vi "ReadAttributeTest.vi"() -> ()   [LabVIEW 2009]
uses:
  tango_lv8/tango_vi.llb/ReadDoubleSpectrumAttribute.vi
  tango_lv8/tango_vi.llb/ReadDoubleScalarAttribute.vi
  tango_lv8/tango_vi.llb/ReadLongScalarAttribute.vi
  tango_lv8/tango_vi.llb/ReadLongSpectrumAttribute.vi
  tango_lv8/tango_vi.llb/ReadShortSpectrumAttribute.vi
  tango_lv8/tango_vi.llb/ReadShortScalarAttribute.vi
  tango_lv8/tango_vi.llb/ReadShortImageAttribute.vi
  tango_lv8/tango_vi.llb/ReadLongImageAttribute.vi
  tango_lv8/tango_vi.llb/ReadDoubleImageAttribute.vi
  tango_lv8/tango_vi.llb/ReadStringAttribute.vi
panel:
  out "?":string
  out "?":bool
  out "?":string
  out "?":bool
  out "?":string
  out "scalar attr. value 3":i16(graph)
  out "spectrum attr. value 3":i16[](graph)
  out "?":bool
  out "?":string
  out "image attr. value":i16[][](graph)
  out "?":bool
  out "?":string
  out "image attr. value":i32[][](graph)
  out "?":bool
  out "?":string
  out "?":bool
  out "?":string
  out "scalar attr. value 2":i32(graph)
  out "spectrum attr. value 2":i32[](graph)
  out "?":bool
  out "?":string
  out "?":dbl(graph)
  out "?":bool
  out "?":string
  out "?":bool
  out "?":string
  out "?":bool
  out "image attr. value":dbl[][](graph)
  out "?":dbl[](graph)
  out "?":string
  in  "<TangoTest> device name":string="tango/tangotest/1"
  # "TANGO  Binding for LabVIEW - ReadAttribute example"
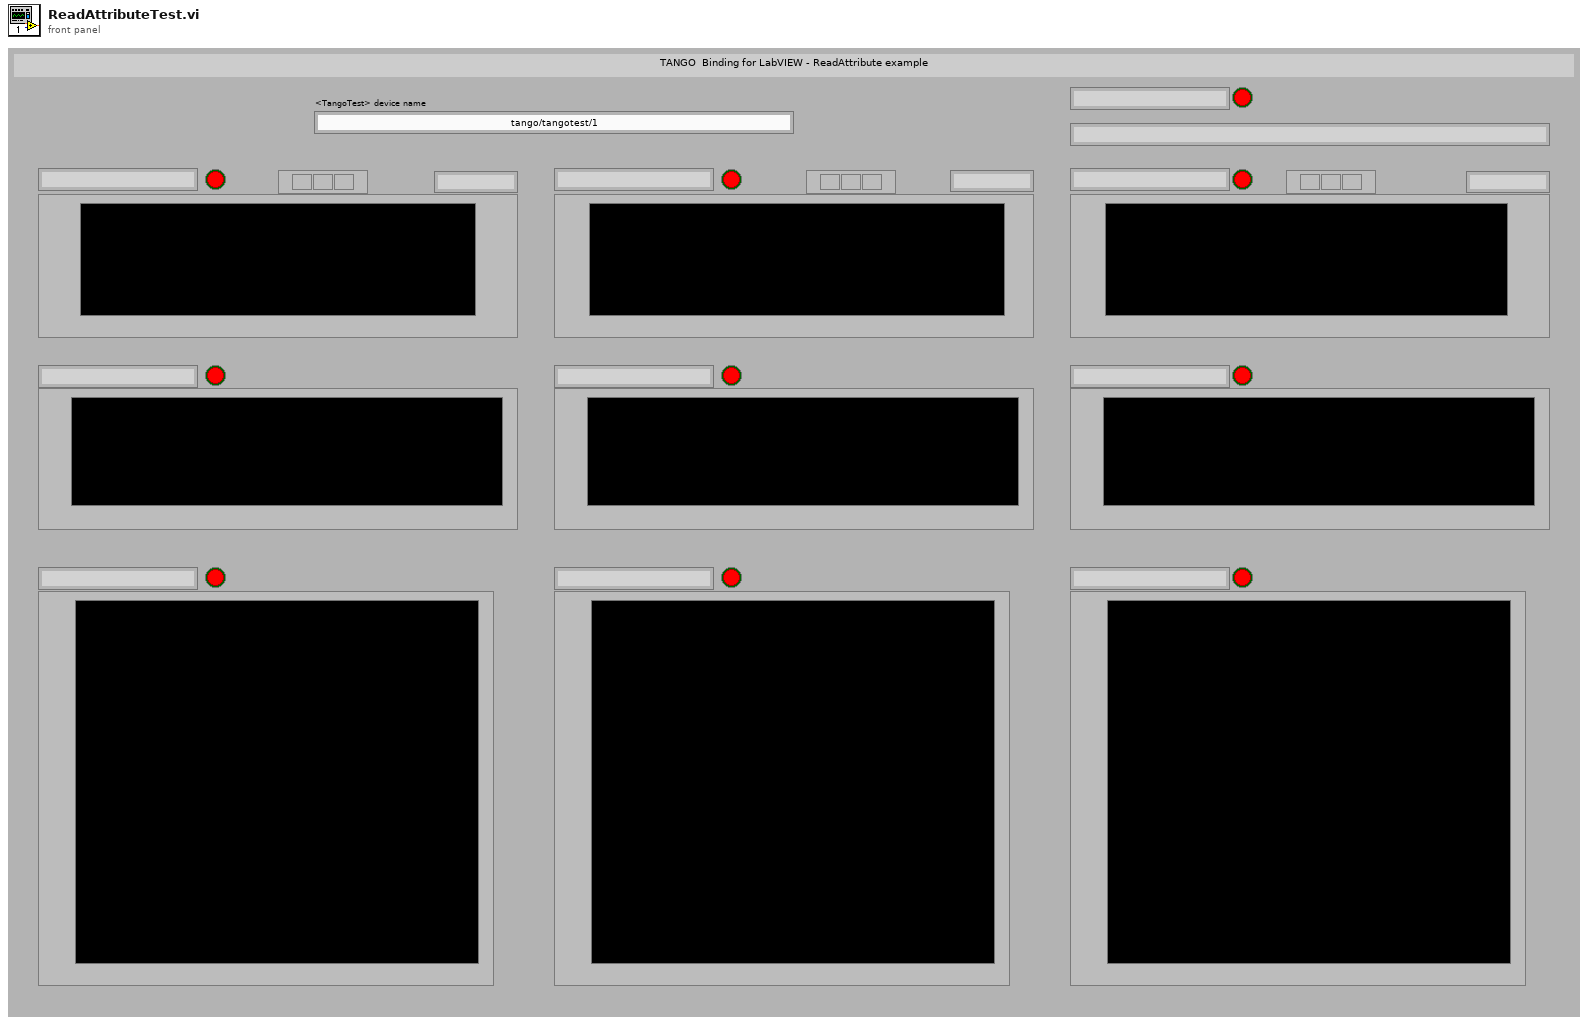
[diagram p1: front panel]
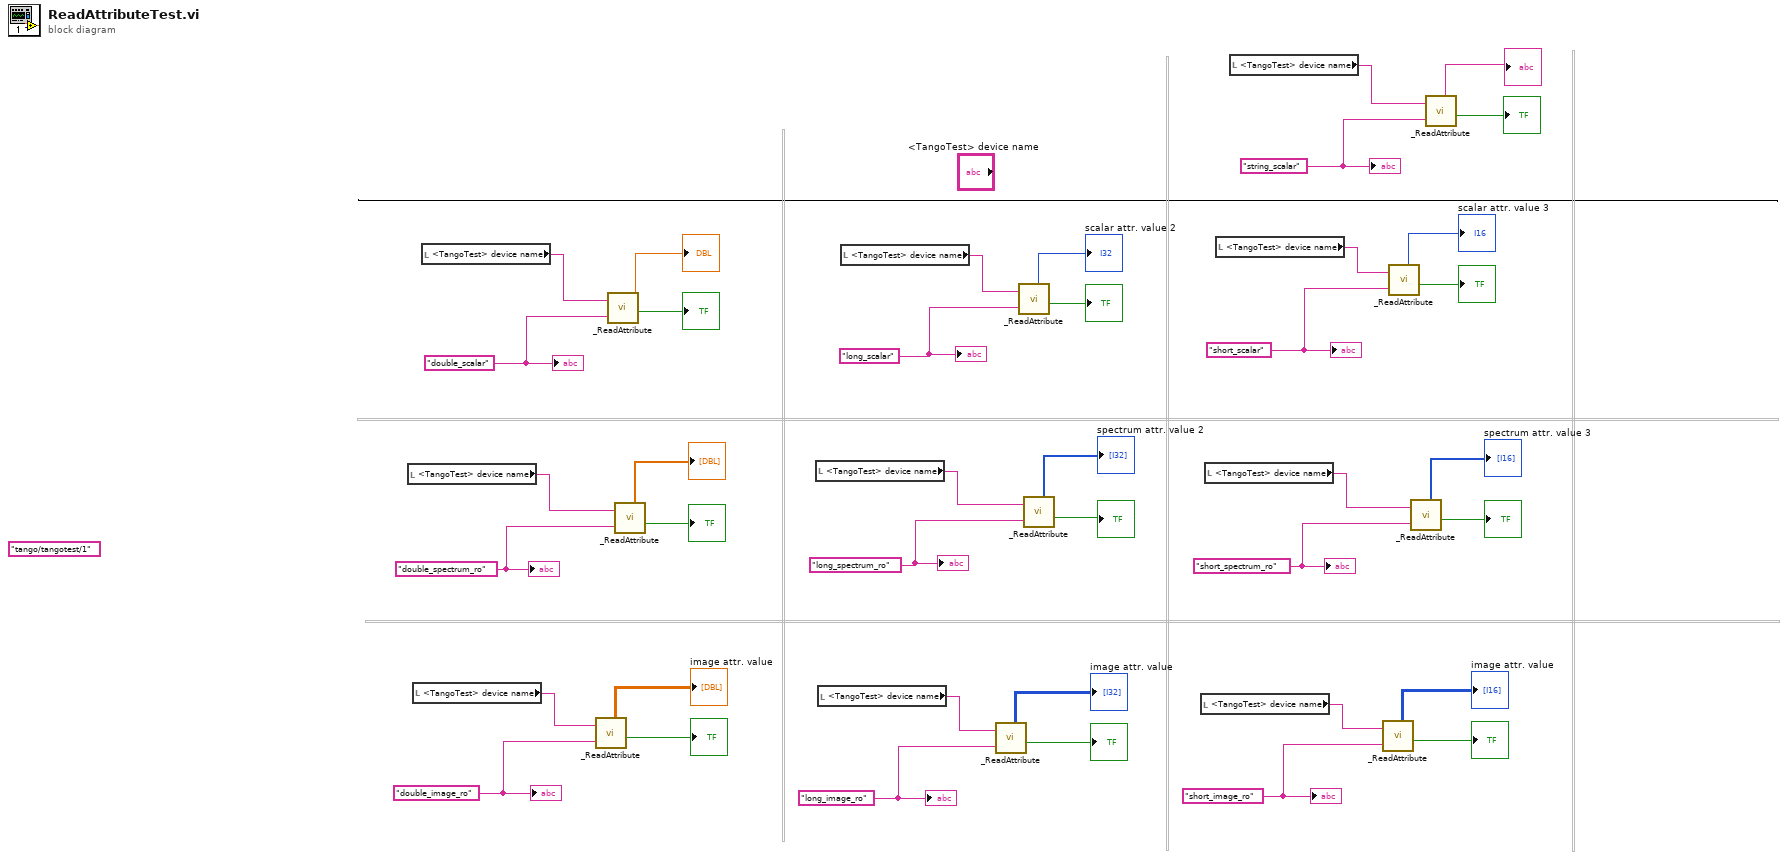
[diagram p0: block diagram]
diagram:
  (unwired) "tango/tangotest/1" ("<TangoTest> device name")
  w11 = "string_scalar"
  w22 = "short_scalar"
  w24 = "short_spectrum_ro"
  w26 = "short_image_ro" ("attr_name")
  w28 = "long_image_ro" ("attr_name")
  w31 = "long_scalar"
  w34 = "long_spectrum_ro"
  w36 = "double_image_ro" ("attr_name")
  w2 = "double_scalar"
  w40 = "double_spectrum_ro"
  n1 = local read "<TangoTest> device name"() -> (w20:string)
  n2 = local read "<TangoTest> device name"() -> (w19:string)
  n3 = local read "<TangoTest> device name"() -> (w13:string)
  n4 = call-poly "_ReadAttribute.vi"("device name"=w19, "attribute name"=w36) -> ("value"=→"image attr. value":dbl[][], "success"=→"?":bool)  [unwired: 4 out]
  n5 = call-poly "_ReadAttribute.vi"("device name"=w13, "attribute name"=w2) -> ("timestamp"=→"?":dbl, "success"=→"?":bool)  [unwired: 4 out]
  n6 = call-poly "_ReadAttribute.vi"("device name"=w20, "attribute name"=w40) -> ("value"=→"?":dbl[], "success"=→"?":bool)  [unwired: 4 out]
  n7 = local read "<TangoTest> device name"() -> (w18:string)
  n8 = local read "<TangoTest> device name"() -> (w17:string)
  n9 = local read "<TangoTest> device name"() -> (w12:string)
  n10 = call-poly "_ReadAttribute.vi"("device name"=w17, "attribute name"=w28) -> ("value"=→"image attr. value":i32[][], "success"=→"?":bool)  [unwired: 4 out]
  n11 = call-poly "_ReadAttribute.vi"("device name"=w12, "attribute name"=w31) -> ("value"=→"scalar attr. value 2":i32, "success"=→"?":bool)  [unwired: 4 out]
  n12 = call-poly "_ReadAttribute.vi"("device name"=w18, "attribute name"=w34) -> ("value"=→"spectrum attr. value 2":i32[], "success"=→"?":bool)  [unwired: 4 out]
  n13 = local read "<TangoTest> device name"() -> (w16:string)
  n14 = local read "<TangoTest> device name"() -> (w15:string)
  n15 = local read "<TangoTest> device name"() -> (w14:string)
  n16 = local read "<TangoTest> device name"() -> (w8:string)
  n17 = call-poly "_ReadAttribute.vi"("device name"=w16, "attribute name"=w26) -> ("value"=→"image attr. value":i16[][], "success"=→"?":bool)  [unwired: 4 out]
  n18 = call-poly "_ReadAttribute.vi"("device name"=w14, "attribute name"=w22) -> ("value"=→"scalar attr. value 3":i16, "success"=→"?":bool)  [unwired: 4 out]
  n19 = call-poly "_ReadAttribute.vi"("device name"=w15, "attribute name"=w24) -> ("value"=→"spectrum attr. value 3":i16[], "success"=→"?":bool)  [unwired: 4 out]
  n20 = call-poly "_ReadAttribute.vi"("device name"=w8, "attribute name"=w11) -> ("value"=→"?":string, "success"=→"?":bool)  [unwired: 4 out]
  "?" <- w40
  "?" <- w2
  "?" <- w36
  "?" <- w34
  "?" <- w31
  "?" <- w28
  "?" <- w26
  "?" <- w24
  "?" <- w22
  "?" <- w11
